vi "IV-Trace_v1.03.vi"() -> ()   [LabVIEW 2014]
doc: "This example shows how to configure a measurement and take a reading."
uses:
  <instrlib>/Keithley 24XX/Public/Data/Read (Single Point).vi
  <instrlib>/Keithley 24XX/Keithley 24XX.lvlib
panel:
  out "Analog Data 4":sgl(graph)
  out "Analog Data 3":sgl(graph)
  in  "loop num":dbl=1.0
  out "Data Resistivity":string
  in  "Data Resistivity":path=path "C:/Users/Administrator/Documents/Device-characterization-setup/IV-Trace/Data/dumb/2015_xx_xx_xxxx_xx_keithley_resistivity_001.txt"
  out "Resistance-Voltage":cluster{sgl[], sgl[]}(graph)
  in  "current multiplier":dbl=1.0
  out "Data IV Keithley":string
  in  "Data IV Keithley":path=path "C:/Users/Administrator/Documents/Device-characterization-setup/IV-Trace/Data/dumb/2015_xx_xx_xxxx_xx_keithley_001.txt"
  out "IV Curve":cluster{sgl[], dbl[]}(graph)
  in  "Stop Voltage/Current":dbl=2.0
  in  "Step":dbl=1.0
  in  "Source Mode  (0: Voltage)":u16(ring) items=["Voltage", "Current"]
  in  "Compliance  Level (0.1)":dbl=1.0
  in  "Start Voltage/Current":dbl
  in  "Enable Resistance Auto Range (T:Enable)":bool
  in  "Enable Current Auto Range (T:Enable)":bool=TRUE
  in  "Enable Voltage Auto Range (T:Enable)":bool
  in  "Resistance Manual Range (1.0)":dbl=1.0
  in  "Current Manual Range (1.0)":dbl=1.0
  in  "Voltage Manual Range (1.0)":dbl=1.0
  out "Resistance":sgl
  out "Current":sgl
  out "Voltage":sgl
  in  "Serial Configuration":T1={"Baud Rate"=9600, "Parity"=0, "Data Bits"=8, "Stop Bits"=10, "Flow Control"=0} {"Flow Control" items=["None", "XON/XOFF", "RTS/CTS", "XON/XOFF & RTS/CTS", "DTR/DSR", "XON/XOFF & DTR/DSR"]; "Stop Bits" items=["1.0"=10, "1.5"=15, "2.0"=20]; "Data Bits" items=["7"=7, "8"=8]; "Parity" items=["None", "Odd", "Even", "Mark", "Space"]; "Baud Rate" items=["300"=300, "600"=600, "1200"=1200, "2400"=2400, "4800"=4800, "9600"=9600, "19200"=19200]}
  in  "VISA resource name":refnum<visa-resource-name>="GPIB9::24::INSTR"
  # "NanoBEEs 2015-IV Tracer v1.0"
  # "Source Settings"
  # "GPIB9::24::INSTR"
  # "Voltage Range Settings"
  # "Current Range Settings"
  # "This multiplies the current value\nwith the number that entered, in order\nto  graph lower current values."
  # "Resistance Range Settings"
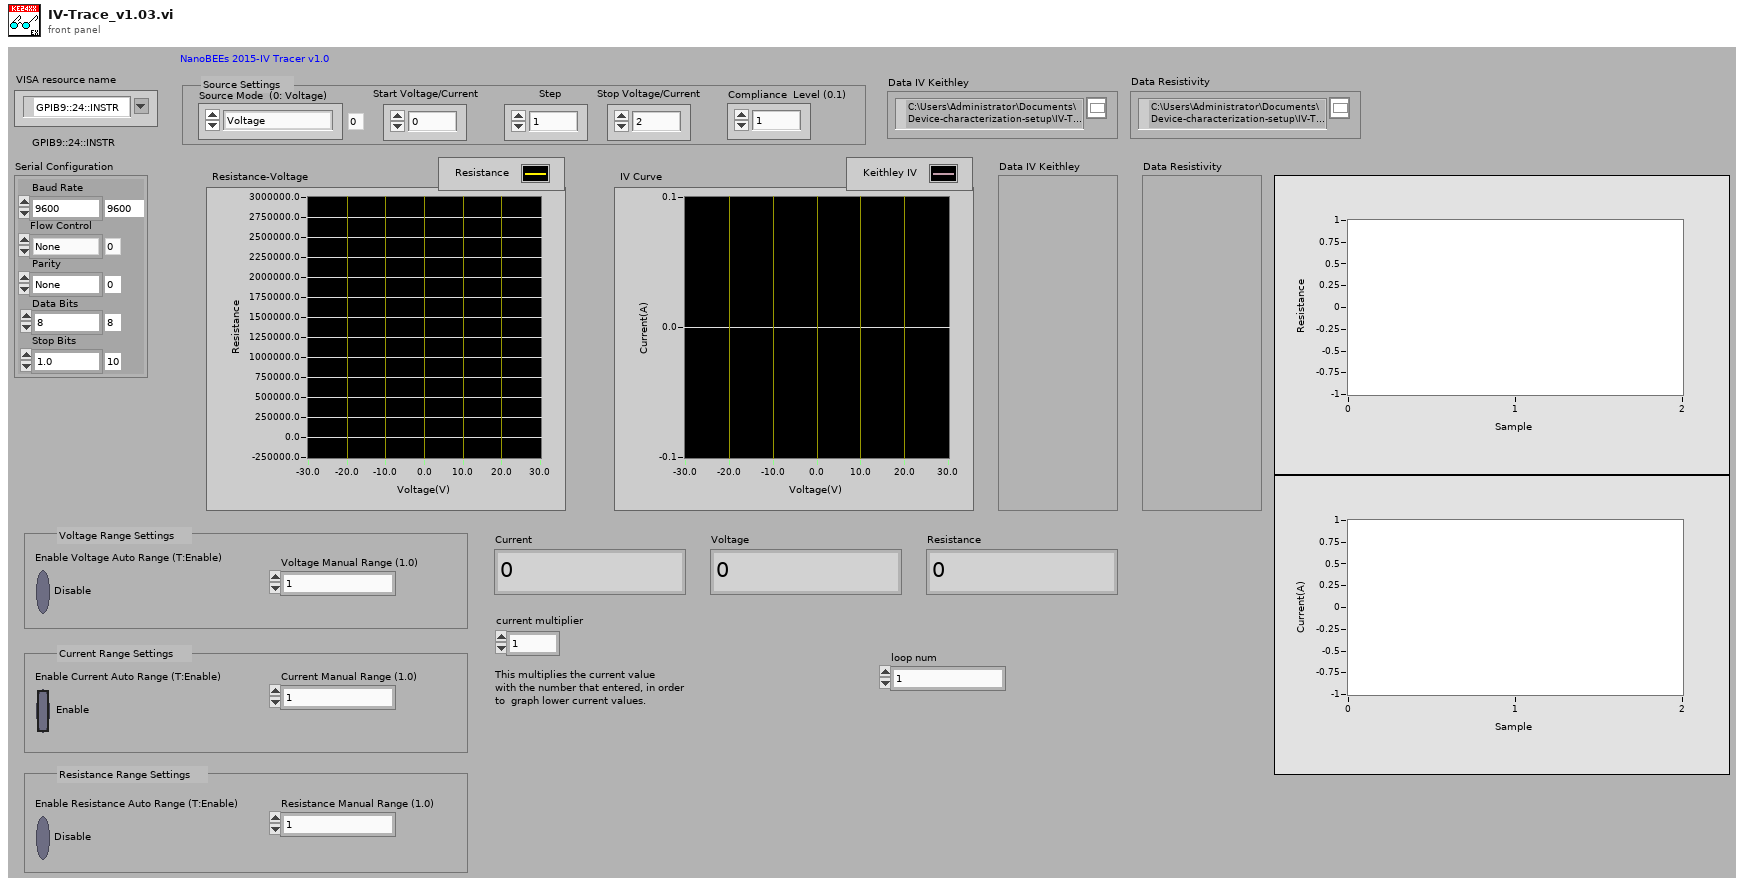
[diagram p1: front panel]
types:
  T1 = cluster{"Baud Rate":u32, "Parity":u16, "Data Bits":u16, "Stop Bits":u16, "Flow Control":u16}
  T2 = enum16{"open", "replace", "create", "open or create", "replace or create", "replace or create with confirmation"}
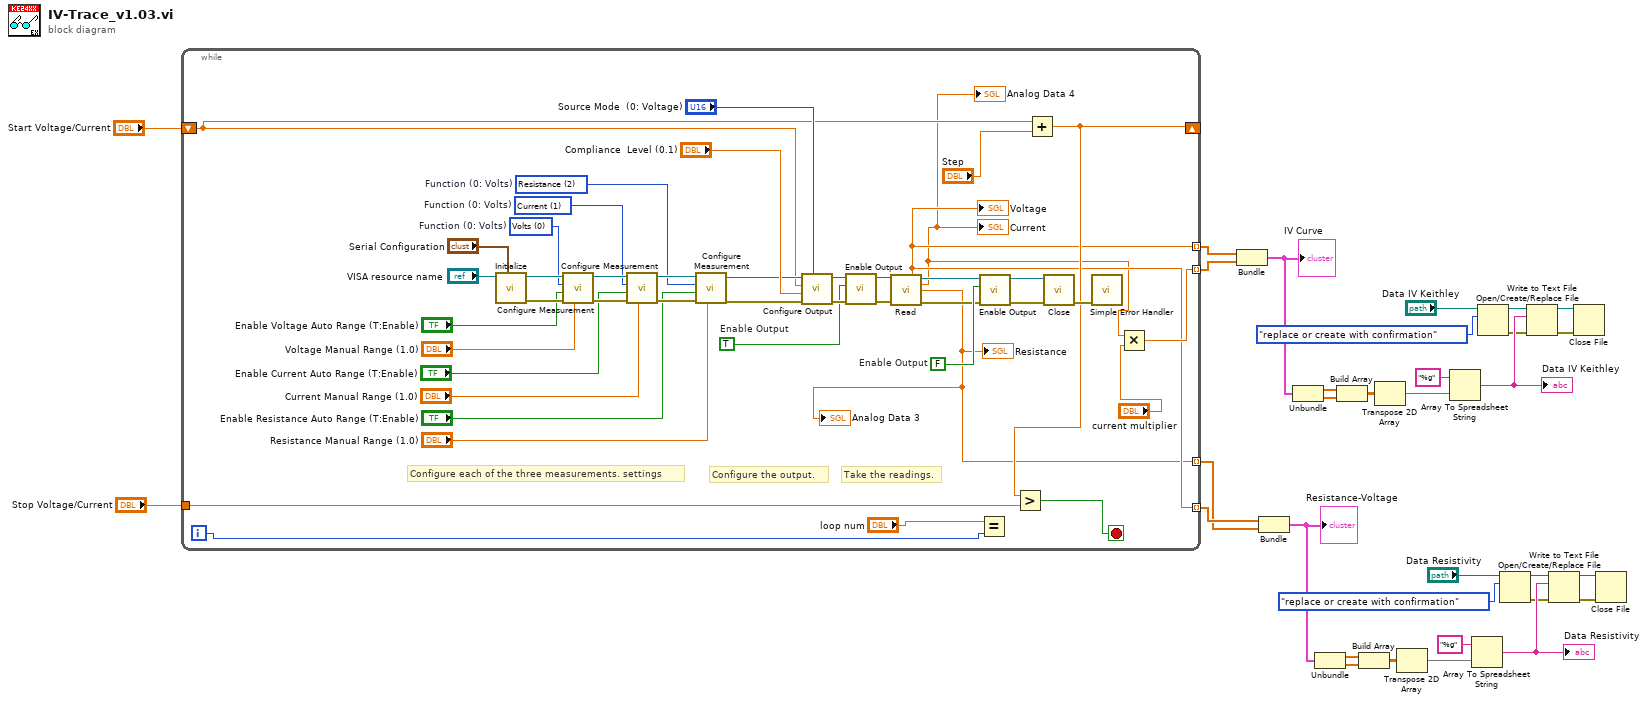
[diagram p0: block diagram]
diagram:
  n1 = while {
    shift-right: [w39] -> _
    shift-left: "Start Voltage/Current" -> [w44]
    tunnel: "Stop Voltage/Current" -> [w42]
    tunnel: [w41] -> w17 mode=indexing
    tunnel: [w38] -> w16 mode=indexing
    tunnel: [w36] -> w1 mode=indexing
    tunnel: [w38] -> w2 mode=indexing
    i -> [w37]
    stop <- w33 stop-if-true
    w48 = TRUE  # Enable Output
    w58 = FALSE  # Enable Output
    w65 = u16 2 items=["Volts", "Current", "Resistance"]  # Function (0: Volts)
    w66 = u16 1 items=["Volts", "Current", "Resistance"]  # Function (0: Volts)
    w67 = u16 0 items=["Volts", "Current", "Resistance"]  # Function (0: Volts)
    # "Take the readings."
    # "Configure the output."
    # "Configure each of the three measurements. settings"
    n2 = call <instrlib>:"Initialize.vi"("Serial Configuration"="Serial Configuration", "VISA resource name"="VISA resource name") -> ("error out"=w72:errorcluster, "VISA resource name out"=w73:refnum<visa-resource-name>)  [unwired: 8 in]
    n3 = call <instrlib>:"Configure Measurement.vi"("Manual Range (1.0)"="Voltage Manual Range (1.0)", "error in (no error)"=w72, "Enable Auto Range (T:Enable)"="Enable Voltage Auto Range (T:Enable)", "Function (0: Volts)"=w67, "VISA resource name"=w73) -> ("error out"=w70:errorcluster, "VISA resource name out"=w71:refnum<visa-resource-name>)  [unwired: 5 in]
    n4 = call <instrlib>:"Configure Measurement.vi"("Manual Range (1.0)"="Current Manual Range (1.0)", "error in (no error)"=w70, "Enable Auto Range (T:Enable)"="Enable Current Auto Range (T:Enable)", "Function (0: Volts)"=w66, "VISA resource name"=w71) -> ("error out"=w69:errorcluster, "VISA resource name out"=w68:refnum<visa-resource-name>)  [unwired: 5 in]
    n5 = call <instrlib>:"Configure Measurement.vi"("Manual Range (1.0)"="Resistance Manual Range (1.0)", "error in (no error)"=w69, "Enable Auto Range (T:Enable)"="Enable Resistance Auto Range (T:Enable)", "Function (0: Volts)"=w65, "VISA resource name"=w68) -> ("error out"=w47:errorcluster, "VISA resource name out"=w46:refnum<visa-resource-name>)  [unwired: 5 in]
    n6 = call <instrlib>:"Configure Output.vi"("Source Mode  (0: Voltage)"="Source Mode  (0: Voltage)", "error in (no error)"=w47, "Compliance  Level (0.1)"="Compliance  Level (0.1)", "Output Level (0)"=w44, "VISA resource name"=w46) -> ("error out"=w49:errorcluster, "VISA resource name out"=w50:refnum<visa-resource-name>)  [unwired: 5 in]
    n7 = call <instrlib>:"Enable Output.vi"("error in (no error)"=w49, "Enable Output (T: Enable)"=w48, "VISA resource name"=w50) -> ("error out"=w52:errorcluster, "VISA resource name out"=w51:refnum<visa-resource-name>)  [unwired: 7 in]
    n8 = call-poly <instrlib>:"Read.vi"("VISA resource name"=w51, "error in (no error)"=w52) -> ("Voltage"=w38:sgl, "VISA resource name out"=w53:refnum<visa-resource-name>, "Current"=w35:sgl, "Resistance"=w36:sgl, "error out"=w54:errorcluster)  [unwired: 7 in, 2 out]
    "Voltage" <- w38
    "Current" <- w35
    "Resistance" <- w36
    "Analog Data 3" <- w36
    "Analog Data 4" <- w35
    n9 = Equal?(x="loop num", y=w37) -> ()  [unwired: 1 out]
    n10 = call <instrlib>:"Enable Output.vi"("error in (no error)"=w54, "Enable Output (T: Enable)"=w58, "VISA resource name"=w53) -> ("error out"=w55:errorcluster, "VISA resource name out"=w56:refnum<visa-resource-name>)  [unwired: 7 in]
    n11 = Add(x=w44, y="Step") -> (x+y=w39:dbl)
    n12 = Greater?(x=w39, y=w42) -> (0:w33:bool)
    n13 = call <instrlib>:"Close.vi"("error in (no error)"=w55, "VISA resource name"=w56) -> ("error out"=w76:errorcluster)  [unwired: 9 in]
    n14 = call <vilib>:"Simple Error Handler.vi"("error in (no error)"=w76) -> ()  [unwired: 4 in, 5 out]
    n15 = Multiply(x=w35, y="current multiplier") -> (x*y=w41:dbl)
  }
  n16 = Bundle(w16, w17) -> (w24:cluster{sgl[], dbl[]})  [unwired: 1 out]
  "IV Curve" <- w24
  n17 = Bundle(w2, w1) -> (w9:cluster{sgl[], sgl[]})  [unwired: 1 out]
  "Resistance-Voltage" <- w9
  n18 = Unbundle(w24) -> (w25:sgl[], w26:dbl[])
  n19 = Unbundle(w9) -> (w10:sgl[], w11:sgl[])
  n20 = Build Array(w25, w26) -> (w27:dbl[][])
  n21 = Build Array(w10, w11) -> (w12:sgl[][])
  n22 = Transpose 2D Array(2D array=w27) -> (transposed array=w29:dbl[][])
  n23 = Transpose 2D Array(2D array=w12) -> (transposed array=w14:sgl[][])
  n24 = Array To Spreadsheet String(array=w29, 3:"%g" ("format string")) -> (spreadsheet string=w30:string)  [unwired: 1 in]
  "Data IV Keithley" <- w30
  n25 = Array To Spreadsheet String(array=w14, 3:"%g" ("format string")) -> (spreadsheet string=w15:string)  [unwired: 1 in]
  "Data Resistivity" <- w15
  n26 = Open/Create/Replace File(file path (use dialog)="Data IV Keithley", operation (0:open)=T2."replace or create with confirmation") -> (refnum out=w23:refnum<file>, error out=w18:errorcluster)  [unwired: 4 in, 1 out]
  n27 = Open/Create/Replace File(file path (use dialog)="Data Resistivity", operation (0:open)=T2."replace or create with confirmation") -> (refnum out=w8:refnum<file>, error out=w3:errorcluster)  [unwired: 4 in, 1 out]
  n28 = Write to Text File(file (use dialog)=w23, text=w30, error in=w18) -> (refnum out=w20:refnum<file>, error out=w19:errorcluster)  [unwired: 2 out]
  n29 = Write to Text File(file (use dialog)=w8, text=w15, error in=w3) -> (refnum out=w5:refnum<file>, error out=w4:errorcluster)  [unwired: 2 out]
  n30 = Close File(refnum=w20, error in=w19) -> ()  [unwired: 2 out]
  n31 = Close File(refnum=w5, error in=w4) -> ()  [unwired: 2 out]
